vi "_Create HTML file and folders.vi"(0 "Menu Launch:App":refnum<vi>, 2 "HTML File Path":path, 5 "Menu Launch:VI":string, 11 "error in (no error)":errorcluster) -> (4 "HTML FIle Path out":path, 15 "error out":errorcluster)   [LabVIEW 2012]
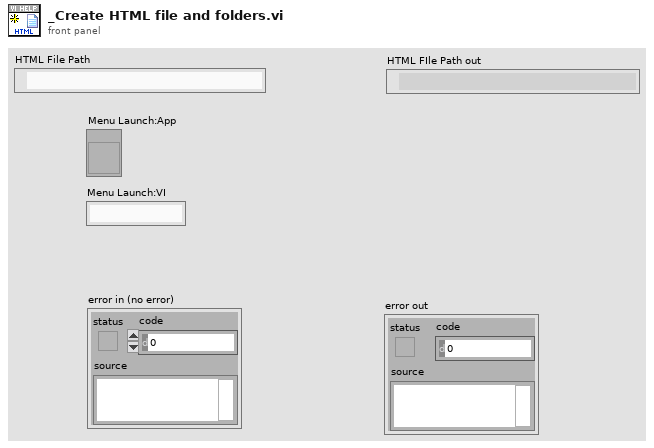
[diagram p1: front panel]
types:
  T1 = enum32{"Custom", "Standard", "Using Panel", "Using SubVI", "Complete"}
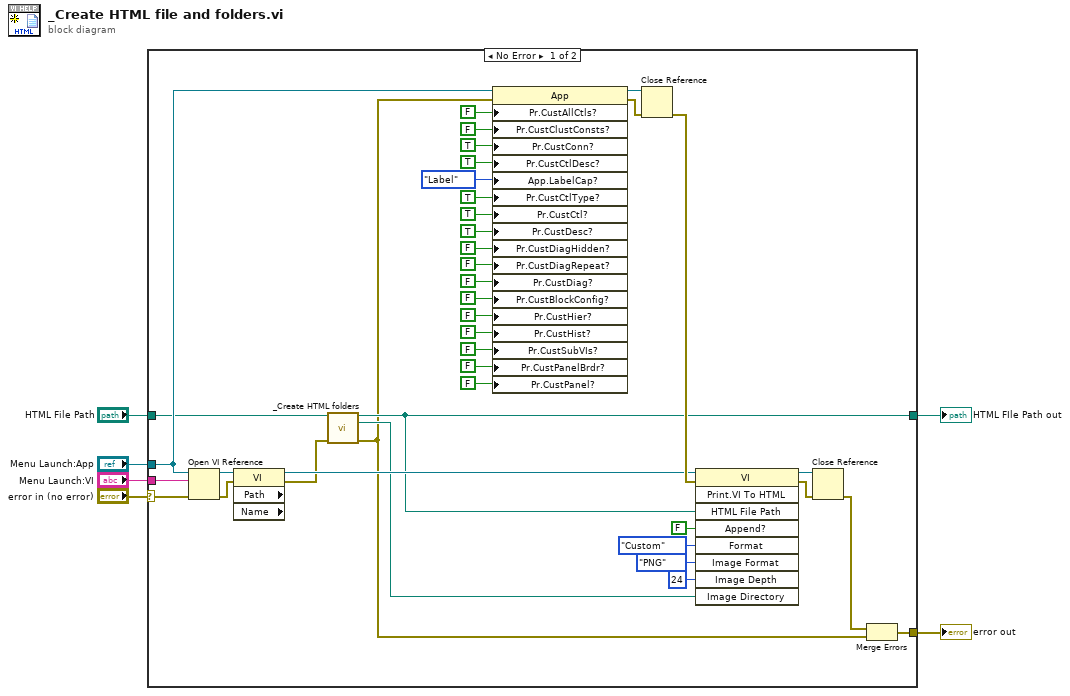
[diagram p0: block diagram]
diagram:
  n1 = case shown="No Error" "error in (no error)" {
    selector: "error in (no error)" -> [w7 w46]
    tunnel: [w19 w46] -> w6
    tunnel: "Menu Launch:VI" -> [w17 _]
    tunnel: "Menu Launch:App" -> [w16 _]
    tunnel: "HTML File Path" -> [w13 w47]
    tunnel: [w11 w47] -> w2
    frame No Error {
      n2 = Open VI Reference(application reference (local)=w16, vi path=w17, error in (no error)=w7) -> (vi reference=w15:refnum<vi>, error out=w14:errorcluster)  [unwired: 3 in]
      n3 = property class="VI" props=["Path", "Name"](reference=w15, error in=w14) -> (reference out=w39:refnum<vi>, error out=w12:errorcluster)  [unwired: 2 out]
      n4 = call "_Create HTML folders.vi"("HTML File Path"=w13, "error in (no error)"=w12) -> ("HTML FIle Path out"=w11:path, "HTML Images Folder"=w10:path, "error out"=w8:errorcluster)  [unwired: 10 in, 1 out]
      n5 = property class="App"(reference=w16, error in=w8, "Pr.CustAllCtls?"=FALSE ("Printing:Custom All Controls?"), "Pr.CustClustConsts?"=FALSE ("Printing:Custom All Controls?"), "Pr.CustConn?"=TRUE ("Printing:Custom Connector?"), "Pr.CustCtlDesc?"=TRUE ("Printing:Custom Control Descriptions?"), "App.LabelCap?"=enum16{"Label", "Caption", "Caption[Label]"}."Label" ("Printing:Custom Control Label/Caption?"), "Pr.CustCtlType?"=TRUE ("Printing:Custom Control Types?"), "Pr.CustCtl?"=TRUE ("Printing:Custom Controls?"), "Pr.CustDesc?"=TRUE ("Printing:Custom Description?"), "Pr.CustDiagHidden?"=FALSE ("Printing:Custom Diagram Hidden?"), "Pr.CustDiagRepeat?"=FALSE ("Printing:Custom Diagram Repeat?"), "Pr.CustDiag?"=FALSE ("Printing:Custom Diagram?"), "Pr.CustBlockConfig?"=FALSE ("Printing:Custom Express VI Configuration?"), "Pr.CustHier?"=FALSE ("Printing:Custom Hierarchy?"), "Pr.CustHist?"=FALSE ("Printing:Custom History?"), "Pr.CustSubVIs?"=FALSE ("Printing:Custom List of SubVIs?"), "Pr.CustPanelBrdr?"=FALSE ("Printing:Custom Panel Border?"), "Pr.CustPanel?"=FALSE ("Printing:Custom Panel?")) -> (reference out=w37:refnum<vi>, error out=w36:errorcluster)
      n6 = Close Reference(reference=w37, error in (no error)=w36) -> (error out=w42:errorcluster)
      n7 = invoke class="VI" method="Print.VI To HTML"(reference=w39, error in=w42, "HTML File Path"=w11, "Append?"=FALSE, "Format"=T1."Custom", "Image Format"=enum32{"PNG", "JPEG", "GIF"}."PNG", "Image Depth"=24, "Image Directory"=w10) -> (reference out=w41:refnum<vi>, error out=w40:errorcluster)  [unwired: 1 in, 7 out]
      n8 = Close Reference(reference=w41, error in (no error)=w40) -> (error out=w9:errorcluster)
      n9 = Merge Errors(w9, w8) -> (w19:errorcluster)
    }
    frame Error {
    }
  }
  "error out" <- w6
  "HTML FIle Path out" <- w2
